vi "ExampleClassDriver.vi"() -> ()   [LabVIEW 2012]
uses:
  ExampleClass.lvclass
panel:
  out "Number":i32
  out "Message":string
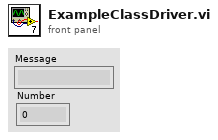
[diagram p1: front panel]
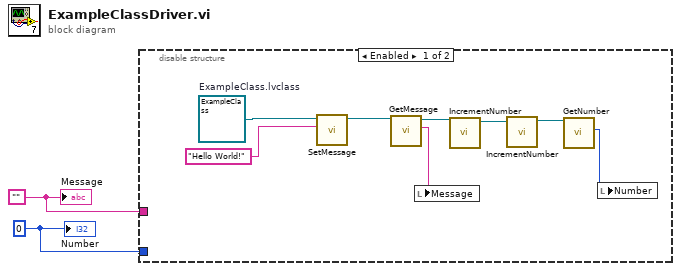
[diagram p0: block diagram]
diagram:
  w2 = 0
  w1 = ""
  n1 = disable-structure shown="Enabled" {
    disable-tunnel: w2 -> [_ _]
    disable-tunnel: w1 -> [_ _]
    frame Enabled {
      w10 = refnum<class "ExampleClass.lvclass"> refnum  # ExampleClass.lvclass
      n2 = call-dynamic "SetMessage.vi"("Message"="Hello World!", "ExampleClass in"=w10) -> ("ExampleClass out"=w8:refnum<class "ExampleClass.lvclass">)  [unwired: 8 in, 1 out]
      n3 = call "GetMessage.vi"("ExampleClass in"=w8) -> ("Message"=w7:string, "ExampleClass out"=w6:refnum<class "ExampleClass.lvclass">)  [unwired: 9 in]
      n4 = local write "Message"(w7) -> ()
      n5 = call "IncrementNumber.vi"("ExampleClass in"=w6) -> ("ExampleClass out"=w5:refnum<class "ExampleClass.lvclass">)  [unwired: 10 in]
      n6 = call "IncrementNumber.vi"("ExampleClass in"=w5) -> ("ExampleClass out"=w4:refnum<class "ExampleClass.lvclass">)  [unwired: 10 in]
      n7 = call-dynamic "GetNumber.vi"("ExampleClass in"=w4) -> ("Number"=w3:i32)  [unwired: 8 in, 2 out]
      n8 = local write "Number"(w3) -> ()
    }
    frame Disabled {
    }
  }
  "Message" <- w1
  "Number" <- w2
